vi "Pre-Install Custom Action.vi"(10 "Variant":variant) -> (0 "error out":errorcluster)   [LabVIEW 2019]
uses:
  <resource>/dialog/lvconfig.llb/LV Config Read String.vi
  <resource>/dialog/lvconfig.llb/LV Config Read Numeric (I32).vi
  <vilib>/Utility/config.llb/Write Key (String).vi
  <vilib>/Utility/config.llb/Write Key (I32).vi
  <vilib>/Utility/config.llb/NI_LVConfig.lvlib
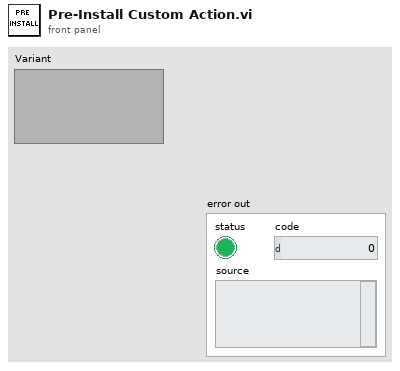
[diagram p1: front panel]
types:
  T1 = typedef "NI_LVConfig.lvlib/Config Data RefNum.ctl" = refnum<k1>
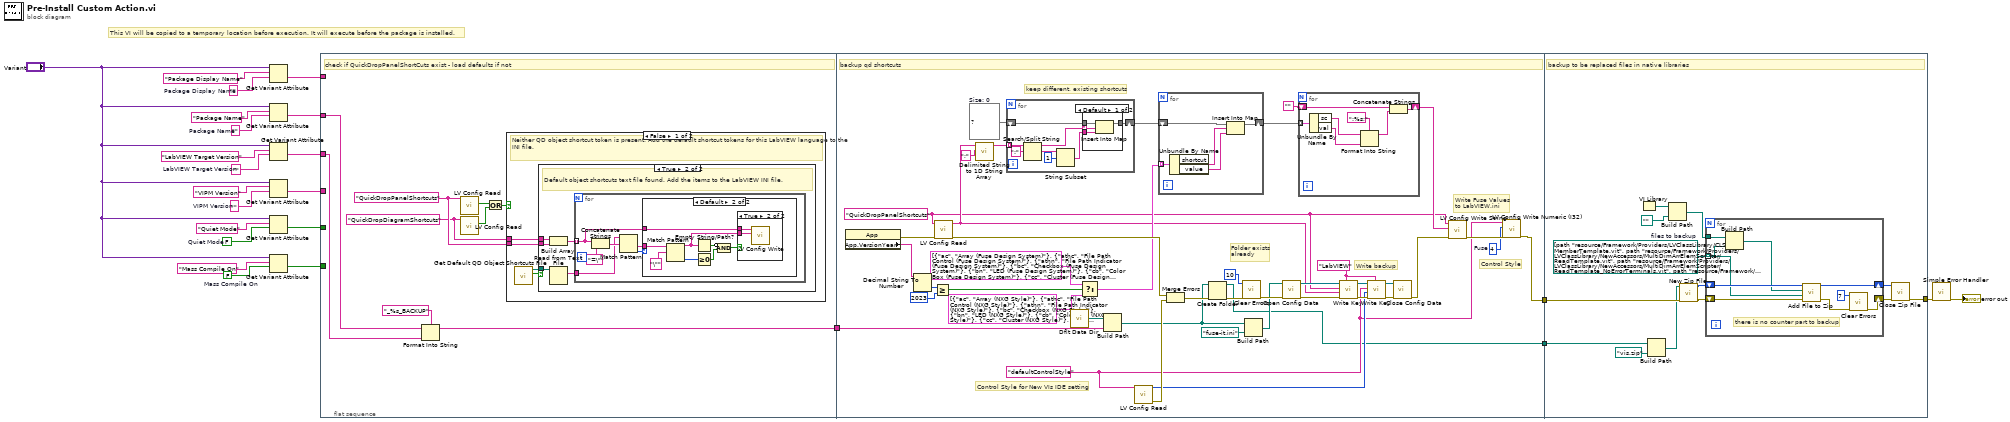
[diagram p0: block diagram]
diagram:
  w3 = FALSE  # Mass Compile On
  w5 = ""  # Package Display Name
  w12 = FALSE  # Quiet Mode
  w15 = ""  # VIPM Version
  w17 = ""  # LabVIEW Target Version
  w19 = ""  # Package Name
  # "This VI will be copied to a temporary location before execution. It will execute before the package is installed."
  n1 = Get Variant Attribute(Variant="Variant", name="Package Display Name", default value (empty Variant)=w5) -> (value=w11:string)  [unwired: 1 in, 3 out]
  n2 = Get Variant Attribute(Variant="Variant", name="Package Name", default value (empty Variant)=w19) -> (value=w10:string)  [unwired: 1 in, 3 out]
  n3 = Get Variant Attribute(Variant="Variant", name="LabVIEW Target Version", default value (empty Variant)=w17) -> (value=w9:string)  [unwired: 1 in, 3 out]
  n4 = Get Variant Attribute(Variant="Variant", name="VIPM Version", default value (empty Variant)=w15) -> (value=w8:string)  [unwired: 1 in, 3 out]
  n5 = Get Variant Attribute(Variant="Variant", name="Quiet Mode", default value (empty Variant)=w12) -> (value=w7:bool)  [unwired: 1 in, 3 out]
  n6 = Get Variant Attribute(Variant="Variant", name="Mass Compile On", default value (empty Variant)=w3) -> (value=w6:bool)  [unwired: 1 in, 3 out]
  n7 = flat-sequence {
    tunnel: w11 -> [_]
    tunnel: w10 -> [w27]
    tunnel: w9 -> [w26]
    tunnel: w8 -> [_]
    tunnel: w7 -> [_]
    tunnel: w6 -> [_]
    tunnel: [w25] -> w2
    tunnel: w2 -> [w73]
    tunnel: [w59] -> w1
    tunnel: [w90] -> w23
    tunnel: [w136] -> w24
    tunnel: w1 -> [w126]
    tunnel: w23 -> [w135]
    frame #0 {
      w32 = "QuickDropDiagramShortcuts" ("Name")
      w33 = "QuickDropPanelShortcuts" ("key")
      # "check if QuickDropPanelShortCuts exist - load defaults if not"
      n8 = Format Into String(format string="_%s_BACKUP", initial string=w27, w26) -> (resulting string=w25:string)  [unwired: 1 in, 1 out]
      n9 = call-poly <resource>:"LV Config Read.vi"("key"=w33) -> ("found?"=w29:bool)  [unwired: 4 in, 2 out]
      n10 = call-poly <resource>:"LV Config Read.vi"("key"=w32) -> ("found?"=w30:bool)  [unwired: 4 in, 2 out]
      n11 = Or(x=w29, y=w30) -> (x .or. y?=w31:bool)
      n12 = case shown="False" w31 {
        tunnel: w32 -> [w37 _]
        tunnel: w33 -> [w36 _]
        frame False {
          # "Neither QD object shortcut token is present. Add the default shortcut tokens for this LabVIEW language to the INI file."
          n13 = call <resource>:"Get Default QD Object Shortcuts File.vi"() -> ("file exists"=w35:bool, "default shortcuts text file"=w34:path)  [unwired: 10 in]
          n14 = case shown="True" w35 {
            tunnel: w34 -> [_ w42]
            tunnel: w37 -> [_ w40]
            tunnel: w36 -> [_ w39]
            frame False {
              # "Default object shortcuts text file does not exist for this language. Do nothing."
            }
            frame True {
              # "Default object shortcuts text file found. Add the items to the LabVIEW INI file."
              n15 = Build Array(w40, w39) -> (w38:string[])
              n16 = Read from Text File(file (use dialog)=w42) -> (text=w41:string)  [unwired: 3 in, 3 out]
              n17 = for {
                tunnel: w41 -> [w44]
                tunnel: w38 -> [w46] mode=indexing
                n18 = Concatenate Strings(w46, "=\"") -> (w45:string)
                n19 = Match Pattern(string=w44, regular expression=w45) -> (after substring=w47:string, offset past match=w43:i32)  [unwired: 1 in, 2 out]
                n20 = case shown="Default" w43 {
                  tunnel: w47 -> [_ w56]
                  tunnel: w46 -> [_ w54]
                  frame -1 {
                  }
                  frame Default {
                    n21 = Match Pattern(string=w56, regular expression="\"") -> (before substring=w53:string, offset past match=w51:i32)  [unwired: 1 in, 2 out]
                    n22 = Empty String/Path?(string/path=w53) -> (empty?=w52:bool)
                    n23 = Greater Or Equal To 0?(x=w51) -> (x >= 0?=w50:bool)
                    n24 = Compound Arithmetic op=AND(invert w52, w50) -> (w49:bool)
                    n25 = case shown="True" w49 {
                      tunnel: w54 -> [_ w58]
                      tunnel: w53 -> [_ w57]
                      frame False {
                      }
                      frame True {
                        n26 = call-poly <resource>:"LV Config Write.vi"("value"=w57, "key"=w58) -> ()  [unwired: 5 in, 1 out]
                      }
                    }
                  }
                }
              }
            }
          }
        }
        frame True {
          # "One or both of the QD object shortcut tokens is already present, don't do anything with loading default shortcuts."
        }
      }
    }
    frame #1 {
      w61 = u32 4  # Fuse
      w62 = "defaultControlStyle" ("key")
      w86 = map{string, string} {}  # Size: 0
      w60 = "QuickDropPanelShortcuts" ("key")
      w66 = "LabVIEW" ("section")
      # "Write backup"
      # "Write Fuse Values\nto LabVIEW.ini"
      # "keep different, existing shortcuts"
      # "Control Style"
      # "Control Style for New VIs IDE setting"
      # "Folder exists\nalready"
      # "backup qd shortcuts"
      n27 = property class="App"() -> (error out=w94:errorcluster, "App.VersionYear"=w79:string)  [unwired: 2 in, 1 out]
      n28 = Decimal String To Number(string=w79) -> (number=w78:i32)  [unwired: 2 in, 1 out]
      n29 = Greater Or Equal?(x=w78, y=2023) -> (x >= y?=w76:bool)
      n30 = call-poly <resource>:"LV Config Read.vi"("error in"=w94, "key"=w60) -> ("error out"=w93:errorcluster, "value"=w65:string)  [unwired: 3 in, 1 out]
      n31 = call <vilib>:"Delimited String to 1D String Array.vi"("delimiter"=";", "delimited string"=w65) -> ("string array"=w87:string[])  [unwired: 9 in]
      n32 = for {
        tunnel: w87 -> [w119] mode=indexing
        shift-right: [w117] -> w85
        shift-left: w86 -> [w118]
        n33 = Search/Split String(string=w119, search string/char (-)=":") -> (substring before match=w116:string, match + rest of string=w115:string)  [unwired: 1 in, 1 out]
        n34 = String Subset(string=w115, offset (0)=1) -> (substring=w114:string)  [unwired: 1 in]
        n35 = case shown="Default" w116 {
          selector: w116 -> [w122 _]
          tunnel: w118 -> [w124 w125]
          tunnel: [w123 w125] -> w117
          tunnel: w114 -> [w121 _]
          frame Default {
            n36 = Insert Into Map(map in=w124, key=w122, value=w121) -> (map out=w123:map{string, string})  [unwired: 2 out]
          }
          frame "" {
          }
        }
      }
      n37 = call <vilib>:"Dflt Data Dir.vi"() -> ("App:Default Data Directory"=w75:path)
      n38 = Select(t=cluster{"shortcut":string, "value":string}[] [{"shortcut"="ac", "value"="Array (Fuse Design System)"}, {"shortcut"="athc", "value"="File Path Control (Fuse Design System)"}, {"shortcut"="athn", "value"="File Path Indicator (Fuse Design System)"}, {"shortcut"="bc", "value"="Checkbox (Fuse Design System)"}, {"shortcut"="bn", "value"="LED (Fuse Design System)"}, {"shortcut"="cb", "value"="Color Box (Fuse Design System)"}, {"shortcut"="cc", "value"="Cluster (Fuse Design System)"}, {"shortcut"="cr", "value"="Control Refnum"}, {"shortcut"="en", "value"="Enum (Fuse Design System)"}, {"shortcut"="erc", "value"="Error In  (Fuse Design System)"}, {"shortcut"="ern", "value"="Error Out (Fuse Design System)"}, {"shortcut"="nc", "value"="Numeric Control (Fuse Design System)"}, {"shortcut"="nn", "value"="Numeric Indicator (Fuse Design System)"}, {"shortcut"="sac", "value"="Select a Control..."}, {"shortcut"="sc", "value"="String Control (Fuse Design System)"}, {"shortcut"="sn", "value"="String Indicator (Fuse Design System)"}, {"shortcut"="vr", "value"="VI Refnum"}, {"shortcut"="wc", "value"="Waveform Chart (Fuse Design System)"}, {"shortcut"="wg", "value"="Waveform Graph (Fuse Design System)"}, {"shortcut"="xg", "value"="XY Graph (Fuse Design System)"}] ("Array"), s=w76, f=cluster{"shortcut":string, "value":string}[] [{"shortcut"="ac", "value"="Array (NXG Style)"}, {"shortcut"="athc", "value"="File Path Control (NXG Style)"}, {"shortcut"="athn", "value"="File Path Indicator (NXG Style)"}, {"shortcut"="bc", "value"="Checkbox (NXG Style)"}, {"shortcut"="bn", "value"="LED (NXG Style)"}, {"shortcut"="cb", "value"="Color Box (NXG Style)"}, {"shortcut"="cc", "value"="Cluster (NXG Style)"}, {"shortcut"="cr", "value"="Control Refnum"}, {"shortcut"="en", "value"="Enum (NXG Style)"}, {"shortcut"="erc", "value"="Error In  (NXG Style)"}, {"shortcut"="ern", "value"="Error Out (NXG Style)"}, {"shortcut"="nc", "value"="Numeric Control (NXG Style)"}, {"shortcut"="nn", "value"="Numeric Indicator (NXG Style)"}, {"shortcut"="sac", "value"="Select a Control..."}, {"shortcut"="sc", "value"="String Control (NXG Style)"}, {"shortcut"="sn", "value"="String Indicator (NXG Style)"}, {"shortcut"="vr", "value"="VI Refnum"}, {"shortcut"="wc", "value"="Waveform Chart (NXG Style)"}, {"shortcut"="wg", "value"="Waveform Graph (NXG Style)"}, {"shortcut"="xg", "value"="XY Graph (NXG Style)"}] ("Array")) -> (s? t:f=w81:cluster{"shortcut":string, "value":string}[])
      n39 = Build Path(base path=w75, name or relative path=w73) -> (appended path=w67:path)
      n40 = call-poly <resource>:"LV Config Read.vi"("key"=w62) -> ("error out"=w92:errorcluster, "value"=w64:i32)  [unwired: 4 in, 1 out]
      n41 = for {
        tunnel: w81 -> [w110] mode=indexing
        shift-right: [w111] -> w84
        shift-left: w85 -> [w112]
        n42 = Unbundle By Name(w110) -> ("shortcut"=w109:string, "value"=w108:string)
        n43 = Insert Into Map(map in=w112, key=w109, value=w108) -> (map out=w111:map{string, string})  [unwired: 2 out]
      }
      n44 = Merge Errors(w93, w92) -> (w95:errorcluster)
      n45 = Create Folder(path (use dialog)=w67, error in=w95) -> (created path=w59:path, error out=w96:errorcluster)  [unwired: 1 in, 1 out]
      n46 = call <vilib>:"Clear Errors.vi"("error in (no error)"=w96, "specific error code to clear (0: all)"=10) -> ("error out"=w100:errorcluster)  [unwired: 4 in, 1 out]
      n47 = Build Path(base path=w67, name or relative path=path "fuse-it.ini") -> (appended path=w68:path)
      n48 = call <vilib>:"Open Config Data.vi"("error in (no error)"=w100, "configuration file path"=w68) -> ("error out"=w99:errorcluster, "refnum"=w71:T1)  [unwired: 7 in, 1 out]
      n49 = for {
        tunnel: w84 -> [w107] mode=indexing
        shift-right: [w103] -> w63
        shift-left: "" -> [w105]
        n50 = Unbundle By Name(w107) -> ("sc"=w101:string, "val"=w102:string)
        n51 = Format Into String(format string=":%s;", initial string=w101, w102) -> (resulting string=w104:string)  [unwired: 1 in, 1 out]
        n52 = Concatenate Strings(w105, w104) -> (w103:string)
      }
      n53 = call-poly <vilib>:"Write Key.vi"("section"=w66, "error in (no error)"=w99, "value"=w65, "key"=w60, "refnum"=w71) -> ("error out"=w98:errorcluster, "refnum out"=w70:T1)  [unwired: 4 in, 1 out]
      n54 = call-poly <vilib>:"Write Key.vi"("section"=w66, "error in (no error)"=w98, "value"=w64, "key"=w62, "refnum"=w70) -> ("error out"=w97:errorcluster, "refnum out"=w69:T1)  [unwired: 4 in, 1 out]
      n55 = call <vilib>:"Close Config Data.vi"("error in (no error)"=w97, "refnum"=w69) -> ("error out"=w91:errorcluster)  [unwired: 8 in, 1 out]
      n56 = call <resource>:"LV Config Write String.vi"("error in (no error)"=w91, "value"=w63, "key"=w60) -> ("error out"=w89:errorcluster)  [unwired: 4 in]
      n57 = call <resource>:"LV Config Write Numeric (I32).vi"("error in (no error)"=w89, "value"=w61, "key"=w62) -> ("error out"=w90:errorcluster)  [unwired: 4 in]
    }
    frame #2 {
      w127 = path[] [path "resource/Framework/Providers/LVClassLibrary/CLSUIP_MemberTemplate.vit", path "resource/Framework/Providers/LVClassLibrary/NewAccessors/MultiDimArrElemScripter/ReadTemplate.vit", path "resource/Framework/Providers/LVClassLibrary/NewAccessors/MultiDimArrElemScripter/ReadTemplate_NoErrorTerminals.vit", path "resource/Framework/Providers/LVClassLibrary/NewAccessors/MultiDimArrElemScripter/WriteTemplate.vit", path "resource/Framework/Providers/LVClassLibrary/NewAccessors/MultiDimArrElemScripter/WriteTemplate_NoErrorTerminals.vit", path "resource/Framework/Providers/LVClassLibrary/NewAccessors/BaseAccessorScripter/ReadTemplate.vit", path "resource/Framework/Providers/LVClassLibrary/NewAccessors/BaseAccessorScripter/ReadTemplate_NoErrorTerminals.vit", path "resource/Framework/Providers/LVClassLibrary/NewAccessors/BaseAccessorScripter/WriteTemplate.vit", path "resource/Framework/Providers/LVClassLibrary/NewAccessors/BaseAccessorScripter/WriteTemplate_NoErrorTerminals.vit", path "resource/Framework/Providers/LVClassLibrary/NewAccessors/ArrayElementScripter/ReadTemplate.vit", path "resource/Framework/Providers/LVClassLibrary/NewAccessors/ArrayElementScripter/ReadTemplate_NoErrorTerminals.vit", path "resource/Framework/Providers/LVClassLibrary/NewAccessors/ArrayElementScripter/WriteTemplate.vit", path "resource/Framework/Providers/LVClassLibrary/NewAccessors/ArrayElementScripter/WriteTemplate_NoErrorTerminals.vit"]  # files to backup
      # "backup to be replaced files in native libraries"
      n58 = VI Library() -> (path=w132:path)
      n59 = Build Path(base path=w126, name or relative path=path "vis.zip") -> (appended path=w128:path)
      n60 = Build Path(base path=w132, name or relative path=path "..") -> (appended path=w130:path)
      n61 = call <vilib>:"New Zip File.vi"("error in (no error)"=w135, "target"=w128) -> ("error out"=w138:errorcluster, "zip file out"=w134:i64)  [unwired: 3 in, 1 out]
      n62 = for {
        tunnel: w127 -> [w139] mode=indexing
        shift-right: [w145] -> w137
        shift-left: w138 -> [w146]
        shift-right: [w143] -> w133
        shift-left: w134 -> [w144]
        tunnel: w130 -> [w140]
        # "there is no counter part to backup"
        n63 = Build Path(base path=w140, name or relative path=w139) -> (appended path=w142:path)
        n64 = call <vilib>:"Add File to Zip.vi"("error in (no error)"=w146, "destination path in zip"=w139, "source file path"=w142, "zip file in"=w144) -> ("error out"=w147:errorcluster, "zip file out"=w143:i64)  [unwired: 6 in]
        n65 = call <vilib>:"Clear Errors.vi"("error in (no error)"=w147, "specific error code to clear (0: all)"=7) -> ("error out"=w145:errorcluster)  [unwired: 4 in, 1 out]
      }
      n66 = call <vilib>:"Close Zip File.vi"("error in (no error)"=w137, "zip file in"=w133) -> ("error out"=w136:errorcluster)  [unwired: 5 in]
    }
  }
  n67 = call <vilib>:"Simple Error Handler.vi"("error in (no error)"=w24) -> ("error out"=→"error out":errorcluster)  [unwired: 4 in, 4 out]
